vi "testing sector pixel v2.vi"(10 "Sector Parameters Right":T2={"Start Angle"=0.13543701171875, "End Angle"=0.3045654296875, "Inner Radius"=309, "Outter Radius"=405, "Hinge X"=947, "Hinge Y"=829, "NumWingSectors"=8}, 11 "Sector Parameters Left":T2={"Start Angle"=0.6541748046875, "End Angle"=0.856201171875, "Inner Radius"=309, "Outter Radius"=405, "Hinge X"=947, "Hinge Y"=829, "NumWingSectors"=8}) -> ()   [LabVIEW 2013]
uses:
  Sector/Accumulate/Sector Parameter Cluster.ctl
  Sector/Accumulate/Single Sector Pixel Cluster.ctl
  <vilib>/Platform/TimedLoop/XDataNode/timing_clust.ctl
  <vilib>/Platform/TimedLoop/XDataNode/nitl_modes.ctl
  <vilib>/Platform/TimedLoop/XDataNode/wakeup.ctl
  Globals/Update Current Pixel Locations Enum.ctl
  <vilib>/rvi/Emulation/niFpgaSctlEmulationGetInTimedLoop.vi
  <vilib>/rvi/Emulation/niFpgaEmulationReportErrorSimple.vi
  <vilib>/rvi/Emulation/niFpgaGetClockAttributes.vi
  <vilib>/rvi/Emulation/niFpgaCriticalErrorInLSC.vi
  Globals/Pixel Location Global.vi
  <vilib>/Platform/TimedLoop/XDataNode/XDataNode.xnode
  FPGA Image Processing.lvlib
  <vilib>/Platform/TimedLoop/XDataNode/XDNodeRunTimeDep.lvlib
panel:
  in  "stop":bool
  out "Pixel 8":T1
  out "Pixel 7":T1
  out "Pixel 6":T1
  out "Pixel 5":T1
  out "Pixel 4":T1
  out "Pixel 3":T1
  out "Pixel 2":T1
  out "Pixel 1":T1
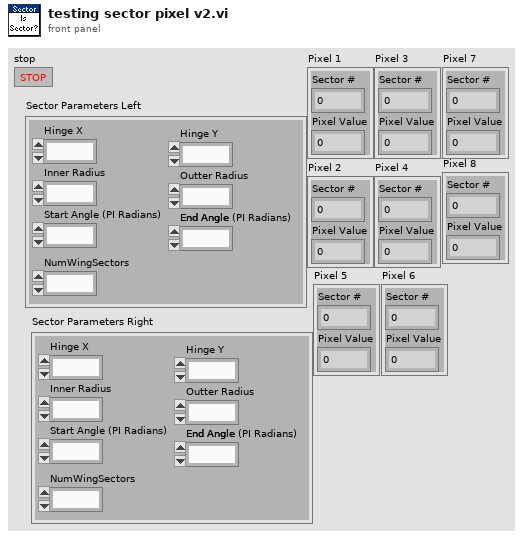
[diagram p1: front panel]
types:
  T1 = typedef "Single Sector Pixel Cluster.ctl" = cluster{"Sector #":u8, "Pixel Value":u8}
  T2 = typedef "Sector Parameter Cluster.ctl" = cluster{"Start Angle":fxp<+,17,3>, "End Angle":fxp<+,17,3>, "Inner Radius":u16, "Outter Radius":u16, "Hinge X":u16, "Hinge Y":u16, "NumWingSectors":u8}
  T3 = typedef "XDNodeRunTimeDep.lvlib/timing_clust.ctl" = cluster{"Expected End [f-1]":u64, "Actual End [f-1]":u64, "Finished Late? [f-1]":bool, "Expected End [i-1]":u64, "Actual End [i-1]":u64, "Finished Late? [i-1]":bool, "Expected Start [i]":u64, "Actual Start [i]":u64, "Expected Start [f]":u64, "Actual Start [f]":u64, "Source Name":string, "Structure Name":string, "Period":i64, "Deadline":i64, "Offset":i64, "Start":i64, "Priority":i32, "Timeout":i32, "Mode":T4, "Wakeup Reason":T5, "Error":errorcluster, "Source Type":string, "Secondary Source Type":string, "Global End Time":u64, "Global Start Time":u64, "Frame Duration":u64, "Iteration Duration":u64, "Assigned CPU":i32, "I/O Scan Engine Mode":u32}
  T4 = typedef "XDNodeRunTimeDep.lvlib/nitl_modes.ctl" = enum32{"No Change", "Process missed periods, maintain original phase", "Discard missed periods, maintain original phase", "Process missed periods, ignore original phase", "Discard missed periods, ignore original phase"}
  T5 = typedef "XDNodeRunTimeDep.lvlib/wakeup.ctl" = enum32{"Normal", "Aborted", "Asynchronous wakeup", "Timing source error", "Timed loop error", "Timeout"}
  T6 = typedef "Update Current Pixel Locations Enum.ctl" = enum16{"Reset", "Update"}
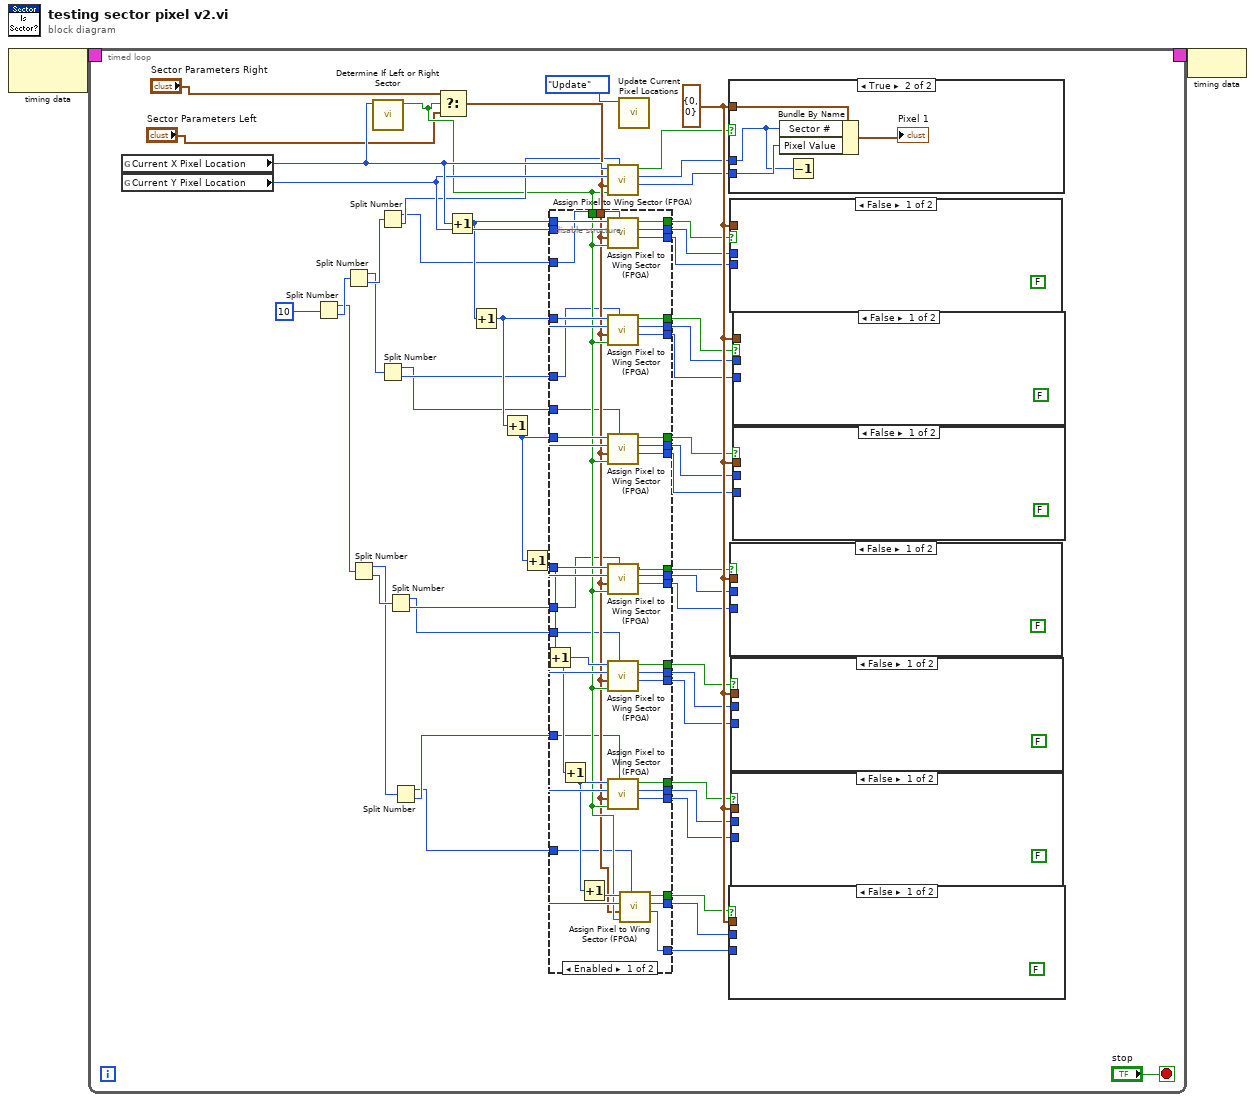
[diagram p0: block diagram]
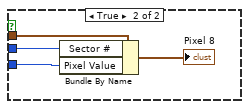
[diagram p3: hidden frame]
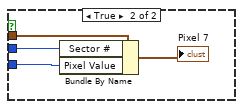
[diagram p4: hidden frame]
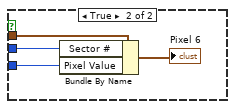
[diagram p5: hidden frame]
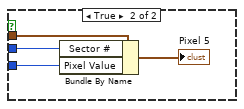
[diagram p6: hidden frame]
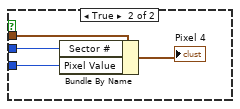
[diagram p7: hidden frame]
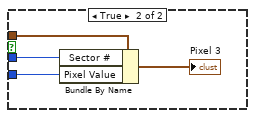
[diagram p8: hidden frame]
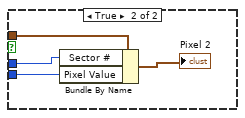
[diagram p9: hidden frame]
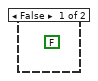
[diagram p10: hidden frame]
diagram:
  n1 = node-c288() -> (w2:T3)  [unwired: 1 in]
  n2 = timed-loop {
    timing: w2 -> [_]
    timing-out: [_] -> w1
    stop <- "stop" stop-if-true
    w41 = T1 {"Sector #"=0, "Pixel Value"=0} ("Single Sector Pixel")
    n3 = global read "Pixel Location Global.vi" "Current X Pixel Location"() -> (w54:u16)
    n4 = global read "Pixel Location Global.vi" "Current Y Pixel Location"() -> (w53:u16)
    n5 = Split Number(x=u64 10 ("Element")) -> (hi(x)=w46:u32, lo(x)=w47:u32)
    n6 = Split Number(x=w47) -> (hi(x)=w44:u16, lo(x)=w45:u16)
    n7 = Split Number(x=w46) -> (hi(x)=w42:u16, lo(x)=w43:u16)
    n8 = call "Determine If Left or Right Sector.vi"("X Pixel Location"=w54) -> ("Right Sector?"=w5:bool)  [unwired: 10 in]
    n9 = Split Number(x=w45) -> (hi(x)=w34:u8, lo(x)=w38:u8)
    n10 = Split Number(x=w44) -> (hi(x)=w24:u8, lo(x)=w28:u8)
    n11 = Split Number(x=w43) -> (hi(x)=w16:u8, lo(x)=w20:u8)
    n12 = Split Number(x=w42) -> (hi(x)=w7:u8, lo(x)=w11:u8)
    n13 = Select(t="Sector Parameters Right", s=w5, f="Sector Parameters Left") -> (s? t:f=w40:T2)
    n14 = Increment(x=w54) -> (x+1=w51:u16)
    n15 = Increment(x=w51) -> (x+1=w50:u16)
    n16 = Increment(x=w50) -> (x+1=w49:u16)
    n17 = Increment(x=w49) -> (x+1=w48:u16)
    n18 = disable-structure shown="Enabled" {
      disable-tunnel: w53 -> [w92 _]
      disable-tunnel: w51 -> [w91 _]
      disable-tunnel: w50 -> [w90 _]
      disable-tunnel: w49 -> [w89 _]
      disable-tunnel: w48 -> [w88 _]
      disable-tunnel: w5 -> [w84 _]
      disable-tunnel: w40 -> [w83 _]
      disable-tunnel: w34 -> [w82 _]
      disable-tunnel: [w81 _] -> w33
      disable-tunnel: [w80 _] -> w32
      disable-tunnel: [w79 _] -> w31
      disable-tunnel: [w78 _] -> w30
      disable-tunnel: [w77 _] -> w29
      disable-tunnel: w28 -> [w76 _]
      disable-tunnel: [w75 _] -> w27
      disable-tunnel: [w74 _] -> w26
      disable-tunnel: [w73 _] -> w25
      disable-tunnel: w24 -> [w72 _]
      disable-tunnel: [w71 _] -> w23
      disable-tunnel: [w70 _] -> w22
      disable-tunnel: [w69 _] -> w21
      disable-tunnel: w20 -> [w68 _]
      disable-tunnel: [w67 _] -> w19
      disable-tunnel: [w66 _] -> w18
      disable-tunnel: [w65 _] -> w17
      disable-tunnel: w16 -> [w64 _]
      disable-tunnel: [w63 _] -> w15
      disable-tunnel: [w62 _] -> w14
      disable-tunnel: [w61 _] -> w13
      disable-tunnel: [w60 _] -> w12
      disable-tunnel: w11 -> [w59 _]
      disable-tunnel: [w58 _] -> w10
      disable-tunnel: [w57 _] -> w9
      disable-tunnel: [w56 _] -> w8
      disable-tunnel: w7 -> [w55 _]
      frame Enabled {
        n19 = Increment(x=w88) -> (x+1=w87:u16)
        n20 = Increment(x=w87) -> (x+1=w86:u16)
        n21 = Increment(x=w86) -> (x+1=w85:u16)
        n22 = call "Assign Pixel to Wing Sector (FPGA).vi"("Pixel Intensity In"=w82, "Right Wing?"=w84, "Sector Parameters"=w83, "Pixel Y"=w92, "Pixel X"=w91) -> ("Pixel Intensity Out"=w79:u8, "sector #"=w80:u8, "output valid"=w81:bool)  [unwired: 3 in]
        n23 = call "Assign Pixel to Wing Sector (FPGA).vi"("Pixel Intensity In"=w76, "Right Wing?"=w84, "Sector Parameters"=w83, "Pixel Y"=w92, "Pixel X"=w90) -> ("Pixel Intensity Out"=w75:u8, "sector #"=w77:u8, "output valid"=w78:bool)  [unwired: 3 in]
        n24 = call "Assign Pixel to Wing Sector (FPGA).vi"("Pixel Intensity In"=w72, "Right Wing?"=w84, "Sector Parameters"=w83, "Pixel Y"=w92, "Pixel X"=w89) -> ("Pixel Intensity Out"=w71:u8, "sector #"=w73:u8, "output valid"=w74:bool)  [unwired: 3 in]
        n25 = call "Assign Pixel to Wing Sector (FPGA).vi"("Pixel Intensity In"=w68, "Right Wing?"=w84, "Sector Parameters"=w83, "Pixel Y"=w92, "Pixel X"=w88) -> ("Pixel Intensity Out"=w67:u8, "sector #"=w69:u8, "output valid"=w70:bool)  [unwired: 3 in]
        n26 = call "Assign Pixel to Wing Sector (FPGA).vi"("Pixel Intensity In"=w64, "Right Wing?"=w84, "Sector Parameters"=w83, "Pixel Y"=w92, "Pixel X"=w87) -> ("Pixel Intensity Out"=w63:u8, "sector #"=w65:u8, "output valid"=w66:bool)  [unwired: 3 in]
        n27 = call "Assign Pixel to Wing Sector (FPGA).vi"("Pixel Intensity In"=w59, "Right Wing?"=w84, "Sector Parameters"=w83, "Pixel Y"=w92, "Pixel X"=w86) -> ("Pixel Intensity Out"=w60:u8, "sector #"=w61:u8, "output valid"=w62:bool)  [unwired: 3 in]
        n28 = call "Assign Pixel to Wing Sector (FPGA).vi"("Pixel Intensity In"=w55, "Right Wing?"=w84, "Sector Parameters"=w83, "Pixel Y"=w92, "Pixel X"=w85) -> ("Pixel Intensity Out"=w56:u8, "sector #"=w57:u8, "output valid"=w58:bool)  [unwired: 3 in]
      }
      frame Disabled {
      }
    }
    n29 = call "Assign Pixel to Wing Sector (FPGA).vi"("Pixel Intensity In"=w38, "Right Wing?"=w5, "Sector Parameters"=w40, "Pixel Y"=w53, "Pixel X"=w54) -> ("Pixel Intensity Out"=w35:u8, "sector #"=w36:u8, "output valid"=w37:bool)  [unwired: 3 in]
    n30 = call "Update Current Pixel Locations.vi"("Operation"=Update_Current_Pixel_Locations_Enum."Update") -> ()  [unwired: 10 in, 1 out]
    n31 = case shown="True" w37 {
      tunnel: w41 -> [_ w124]
      tunnel: w36 -> [_ w121]
      tunnel: w35 -> [_ w122]
      frame False {
        (unwired) FALSE ("Timed Out?")
      }
      frame True {
        n32 = Bundle By Name(cluster=w124, "Sector #"=w121, "Pixel Value"=w122) -> (→"Pixel 1":T1)
        n33 = Decrement(x=w121) -> ()  [unwired: 1 out]
      }
    }
    n34 = case shown="False" w10 {
      tunnel: w41 -> [_ w96]
      tunnel: w9 -> [_ w95]
      tunnel: w8 -> [_ w94]
      frame False {
        (unwired) FALSE ("Timed Out?")
      }
      frame True {
        n35 = Bundle By Name(cluster=w96, "Sector #"=w95, "Pixel Value"=w94) -> (→"Pixel 8":T1)
      }
    }
    n36 = case shown="False" w33 {
      tunnel: w41 -> [_ w120]
      tunnel: w32 -> [_ w118]
      tunnel: w31 -> [_ w117]
      frame False {
        (unwired) FALSE ("Timed Out?")
      }
      frame True {
        n37 = Bundle By Name(cluster=w120, "Sector #"=w118, "Pixel Value"=w117) -> (→"Pixel 2":T1)
      }
    }
    n38 = case shown="False" w22 {
      tunnel: w41 -> [_ w108]
      tunnel: w21 -> [_ w107]
      tunnel: w19 -> [_ w106]
      frame False {
        (unwired) FALSE ("Timed Out?")
      }
      frame True {
        n39 = Bundle By Name(cluster=w108, "Sector #"=w107, "Pixel Value"=w106) -> (→"Pixel 5":T1)
      }
    }
    n40 = case shown="False" w18 {
      tunnel: w41 -> [_ w104]
      tunnel: w17 -> [_ w103]
      tunnel: w15 -> [_ w102]
      frame False {
        (unwired) FALSE ("Timed Out?")
      }
      frame True {
        n41 = Bundle By Name(cluster=w104, "Sector #"=w103, "Pixel Value"=w102) -> (→"Pixel 6":T1)
      }
    }
    n42 = case shown="False" w14 {
      tunnel: w41 -> [_ w100]
      tunnel: w13 -> [_ w99]
      tunnel: w12 -> [_ w98]
      frame False {
        (unwired) FALSE ("Timed Out?")
      }
      frame True {
        n43 = Bundle By Name(cluster=w100, "Sector #"=w99, "Pixel Value"=w98) -> (→"Pixel 7":T1)
      }
    }
    n44 = case shown="False" w30 {
      tunnel: w41 -> [_ w116]
      tunnel: w29 -> [_ w115]
      tunnel: w27 -> [_ w114]
      frame False {
        (unwired) FALSE ("Timed Out?")
      }
      frame True {
        n45 = Bundle By Name(cluster=w116, "Sector #"=w115, "Pixel Value"=w114) -> (→"Pixel 3":T1)
      }
    }
    n46 = case shown="False" w26 {
      tunnel: w41 -> [_ w112]
      tunnel: w25 -> [_ w111]
      tunnel: w23 -> [_ w110]
      frame False {
        (unwired) FALSE ("Timed Out?")
      }
      frame True {
        n47 = Bundle By Name(cluster=w112, "Sector #"=w111, "Pixel Value"=w110) -> (→"Pixel 4":T1)
      }
    }
  }
  n48 = node-c288(w1) -> ()
